vi "update.title.request.vi"(8 "error in":errorcluster, 11 "title":string) -> (0 "error out":errorcluster, 1 "Request":string)   [LabVIEW 2020, in "asset.lvclass"]
uses:
  asset.lvclass
  asset.lvclass/asset.ctl
  116a1f63-1174-4f6f-bedf-07de5800daec.vi
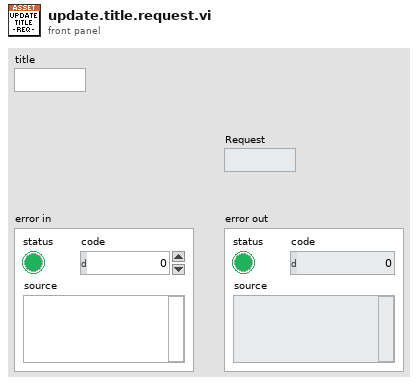
[diagram p1: front panel]
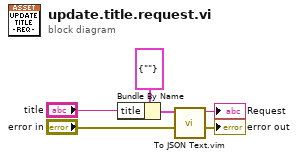
[diagram p0: block diagram]
diagram:
  n1 = Bundle By Name(cluster=cluster{"title":string} {"title"=""}, "title"="title") -> (w5:cluster{"title":string})
  n2 = call "To JSON Text.vim"("error in (no error)"="error in", "Anything"=w5) -> ("error out"=→"error out":errorcluster, "<JSON>"=→"Request":string)  [unwired: 8 in]
